vi "Cfg from FP.vi"(8 "error in (no error)":errorcluster, 11 "Measure Object in":refnum<class "Da Base.lvclass">) -> (0 "error out":errorcluster, 3 "Measure Object out":refnum<class "Da Base.lvclass">)   [LabVIEW 2016, in "Da Base.lvclass"]
uses:
  Da Base.lvclass
  Da Base.lvclass/Da Base.ctl
  Write Configuration.vi
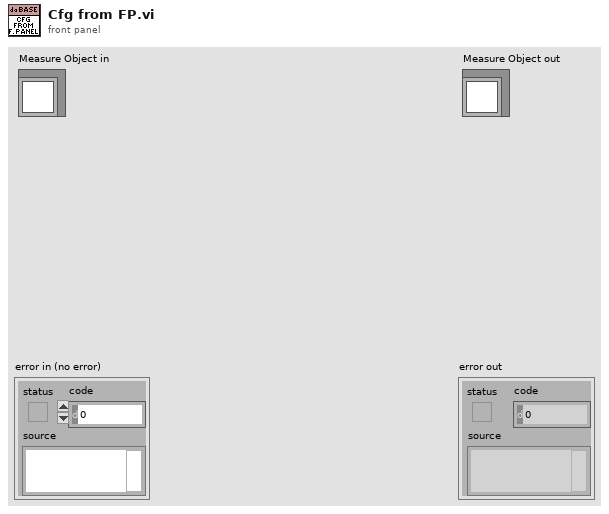
[diagram p1: front panel]
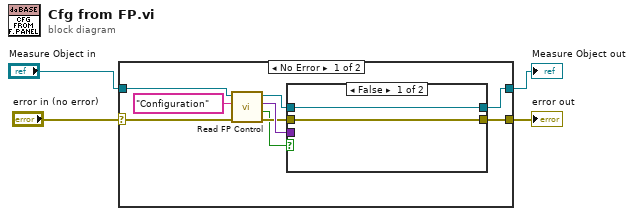
[diagram p0: block diagram]
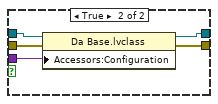
[diagram p2: hidden frame]
diagram:
  n1 = case shown="No Error" "error in (no error)" {
    selector: "error in (no error)" -> [w7 w22]
    tunnel: [w6 w22] -> w3
    tunnel: [w10 w21] -> w1
    tunnel: "Measure Object in" -> [w13 w21]
    frame No Error {
      n2 = call-dynamic "Read FP Control.vi"("error in (no error)"=w7, "Control Name"="Configuration", "Measure Object in"=w13) -> ("error out"=w8:errorcluster, "Present"=w5:bool, "Control Value"=w9:variant, "Measure Object out"=w12:refnum<class "Da Base.lvclass">)  [unwired: 5 in]
      n3 = case shown="False" w5 {
        tunnel: w12 -> [w14 w20]
        tunnel: [w14 w19] -> w10
        tunnel: w9 -> [_ w18]
        tunnel: w8 -> [w15 w17]
        tunnel: [w15 w16] -> w6
        frame False {
        }
        frame True {
          n4 = property class="Da Base.lvclass"(reference=w20, error in=w17, "Accessors:Configuration"=w18) -> (reference out=w19:refnum<class "Da Base.lvclass">, error out=w16:errorcluster)
        }
      }
    }
    frame Error {
    }
  }
  "error out" <- w3
  "Measure Object out" <- w1
